vi "GLB_VAR.vi"() -> ()   [LabVIEW 2024]
uses:
  REF.ctl
  Main Tabs.ctl
  Open Batch Data.ctl
  DM_Data.ctl
  run statistics.ctl
  System settings.ctl
  Printer Message settings.ctl
  ARCH/Message Queue/All Message Queues.ctl
  ARCH/Message Queue/Message Cluster.ctl
  <vilib>/addons/database/Connection.llb/Conn ObjectReference.ctl
  ARCH/Message Queue/Message Queue.lvlib
  <vilib>/addons/database/NI_Database_API.lvlib
panel:
  in  "DB ref":T1
  in  "Printer serials":string[](array[string])
  out "Queues":T2
  out "REF":T3
  out "Batch Running":bool
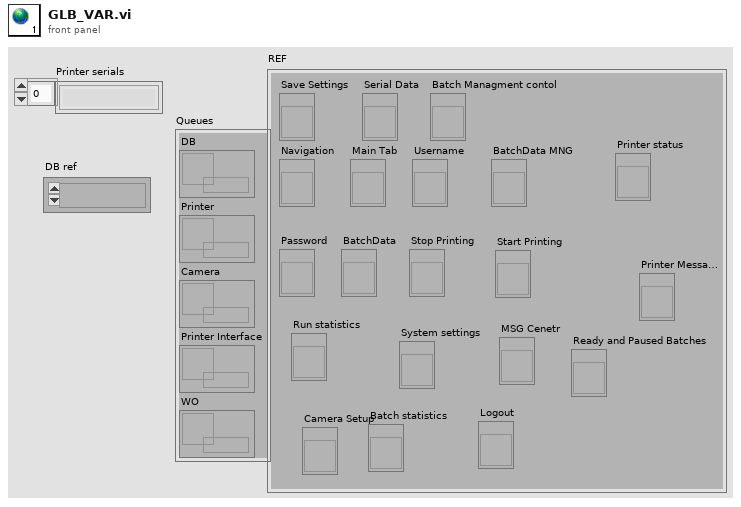
[diagram p1: front panel]
types:
  T1 = typedef "NI_Database_API.lvlib/Conn ObjectReference.ctl" = refnum<k1>
  T2 = typedef "All Message Queues.ctl" = cluster{"DB":refnum<queue>, "Printer":refnum<queue>, "Camera":refnum<queue>, "Printer Interface":refnum<queue>, "WO":refnum<queue>}
  T3 = typedef "REF.ctl" = cluster{"Save Settings":refnum<vi>, "Navigation":refnum<vi>, "Main Tab":refnum<vi>, "Password":refnum<vi>, "BatchData":refnum<vi>, "Serial Data":refnum<vi>, "Username":refnum<vi>, "Stop Printing":refnum<vi>, "Run statistics":refnum<vi>, "System settings":refnum<vi>, "Batch Managment contol":refnum<vi>, "Start Printing":refnum<vi>, "BatchData MNG":refnum<vi>, "MSG Cenetr":refnum<vi>, "Printer status":refnum<vi>, "Printer Message Config":refnum<vi>, "Ready and Paused Batches":refnum<vi>, "Camera Setup":refnum<vi>, "Batch statistics":refnum<vi>, "Logout":refnum<vi>}
diagram:
